vi "Stop FP.vi"(8 "error in":errorcluster, 11 "GUI in":refnum<class "GUI.lvclass">) -> (0 "error out":errorcluster, 3 "GUI out":refnum<class "GUI.lvclass">)   [LabVIEW 2018, in "GUI.lvclass"]
uses:
  GUI.lvclass
  G:/sw_repo/For Builds/Reusable/Observer/Observer.lvclass
  GUI.lvclass/GUI.ctl
  Observer/Observer.lvclass/Observer.ctl
  Data/Data.lvclass
  Observer/Observer.lvclass
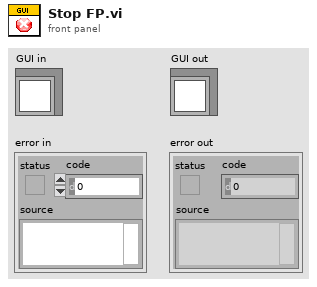
[diagram p1: front panel]
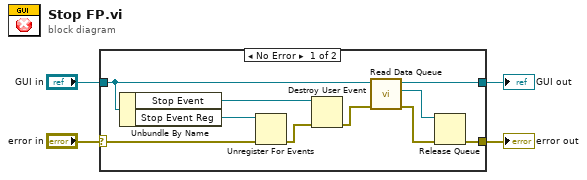
[diagram p0: block diagram]
diagram:
  n1 = case shown="No Error" "error in" {
    selector: "error in" -> [w11 w16]
    tunnel: [w10 w16] -> w3
    tunnel: [w9 w15] -> w1
    tunnel: "GUI in" -> [w5 w15]
    frame No Error {
      n2 = Unbundle By Name(w5) -> ("Stop Event"=w13:refnum<user-event>, "Stop Event Reg"=w14:refnum<event-registration>)
      n3 = Unregister For Events(event registration refnum=w14, error in=w11) -> (error out=w12:errorcluster)
      n4 = Destroy User Event(user event=w13, error in=w12) -> (error out=w6:errorcluster)
      n5 = call "Read Data Queue.vi"("error in (no error)"=w6, "Observer in"=w5) -> ("error out"=w7:errorcluster, "Data Queue"=w8:refnum<queue>, "Observer out"=w9:refnum<class "GUI.lvclass">)  [unwired: 7 in]
      n6 = Release Queue(queue=w8, error in (no error)=w7) -> (error out=w10:errorcluster)  [unwired: 1 in, 2 out]
    }
    frame Error {
    }
  }
  "error out" <- w3
  "GUI out" <- w1
